vi "stage_xy_gui.vi"(10 "enable":refnum<vi>, 11 "conn_xyz_in":T2) -> (0 "position_y":dbl format="%#.3f", 1 "position_x":dbl format="%#.3f", 3 "conn_xyz_out":T1)   [LabVIEW 2014]
uses:
  D:/felipe/Microscope/Software/Tools/Stage_xyz/Dll/Newport.CONEXCC.CommandInterface.dll
  Tools/Stage_xyz/Dll/Newport.CONEXCC.CommandInterface.dll
  <vilib>/Utility/miscctls.llb/LVPointDoubleTypeDef.ctl
  GLOBAL_VAR.vi
panel:
  in  "Tab Control":enum32{"Position", "Status"}(tab)
  in  "y_val":dbl caption="Y:" min=0.0 max=11.0 format="%.3g"
  in  "x_val":dbl caption="X:" min=0.0 max=11.0 format="%.3g"
  out "xy_position":cluster{"X":dbl, "Y":dbl}[](graph)
  in  "stop_move":bool
  out "current_speed_y":dbl=0.4 caption="Y:" min=0.0 max=25.0 format="%#.3f"
  out "state_y":u32 caption="Y:"
  out "state_x":u32 caption="X:"
  out "current_speed_x":dbl=0.4 caption="X:" min=0.0 max=25.0 format="%#.3f"
  # "State :"
  # "Position :"
  # "Speed :"
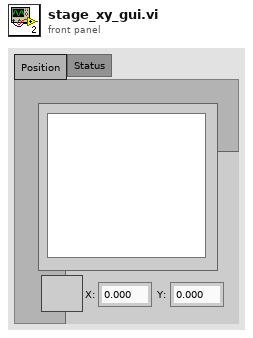
[diagram p1: front panel]
types:
  T1 = cluster{"conn_x_out":refnum<k24>, "conn_y_out":refnum<k24>, "conn_z_out":refnum<k24>}
  T2 = cluster{"conn_x_in":refnum<k24>, "conn_y_in":refnum<k24>, "conn_z_in":refnum<k24>}
  T3 = typedef "LVPointDoubleTypeDef.ctl" = cluster{"X":dbl, "Y":dbl}
  T4 = enum16{"Standby", "Goto", "Stop", "Status", "Goto_z"}
  T5 = cluster{"controllerState":u32, "controllerState":u32, "controllerState":u32}
  T6 = cluster{"Velocity":dbl, "Velocity":dbl, "Velocity":dbl}
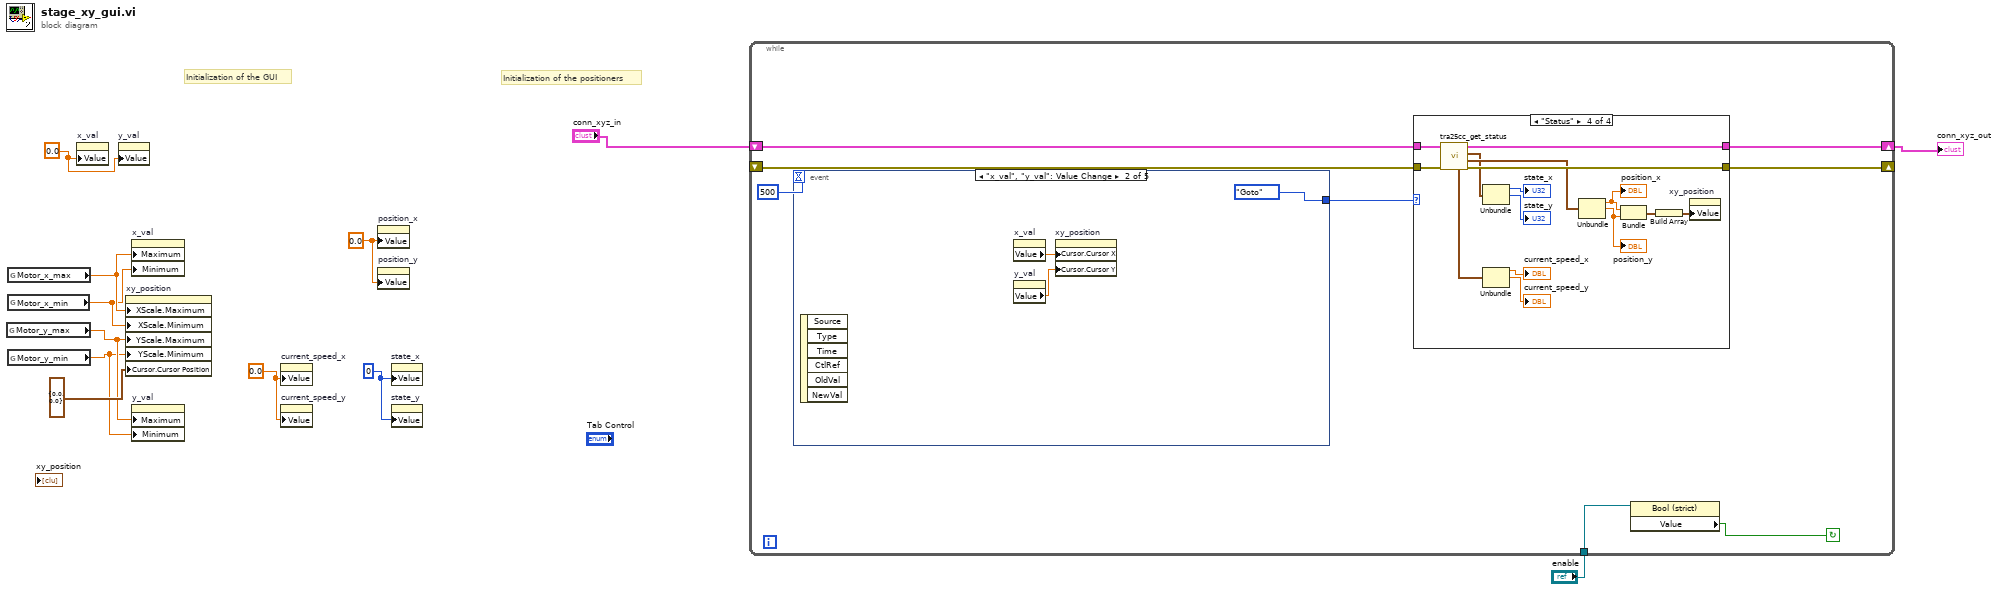
[diagram p0: block diagram]
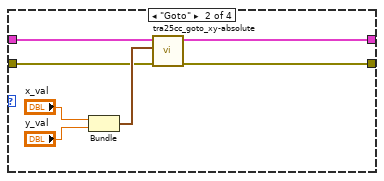
[diagram p3: hidden frame]
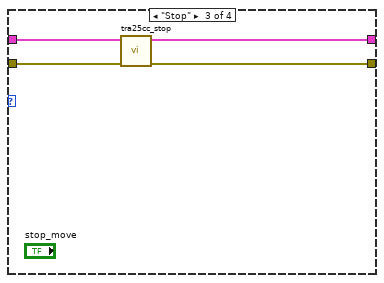
[diagram p4: hidden frame]
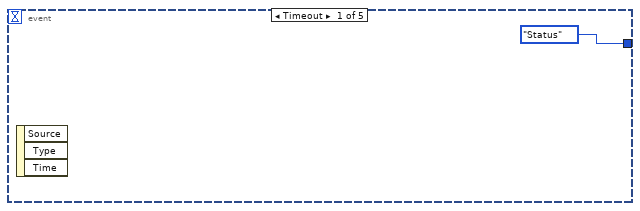
[diagram p5: hidden frame]
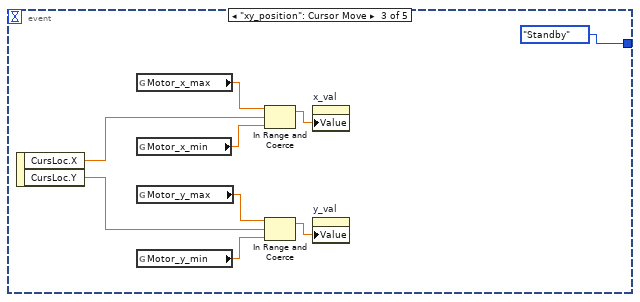
[diagram p6: hidden frame]
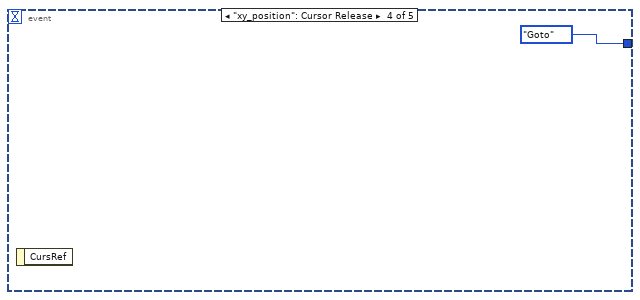
[diagram p7: hidden frame]
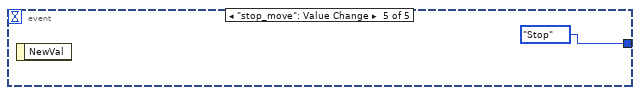
[diagram p8: hidden frame]
diagram:
  w8 = 0.0 ("position_x")
  w9 = u32 0 ("state_x")
  w10 = 0.0 ("current_speed_x")
  w12 = 0.0 ("x_val")
  # "Initialization of the positioners"
  # "Initialization of the GUI"
  n1 = global read "GLOBAL_VAR.vi" "Motor_y_max"() -> (w5:dbl)
  n2 = global read "GLOBAL_VAR.vi" "Motor_x_max"() -> (w7:dbl)
  n3 = global read "GLOBAL_VAR.vi" "Motor_x_min"() -> (w6:dbl)
  n4 = global read "GLOBAL_VAR.vi" "Motor_y_min"() -> (w4:dbl)
  n5 = property on="x_val" class="DigNum (strict)"("Value"=w12) -> ()  [unwired: 2 in, 2 out]
  n6 = property on="y_val" class="DigNum (strict)"("Value"=w12) -> ()  [unwired: 2 in, 2 out]
  n7 = property on="xy_position" class="XYGraph (strict)"("XScale.Maximum"=w7, "XScale.Minimum"=w6, "YScale.Maximum"=w5, "YScale.Minimum"=w4, "Cursor.Cursor Position"=T3 {"X"=0.0, "Y"=0.0}) -> ()  [unwired: 2 in, 2 out]
  n8 = property on="x_val" class="DigNum (strict)"("Maximum"=w7, "Minimum"=w6) -> ()  [unwired: 2 in, 2 out]
  n9 = property on="y_val" class="DigNum (strict)"("Maximum"=w5, "Minimum"=w4) -> ()  [unwired: 2 in, 2 out]
  n10 = property on="current_speed_x" class="DigNum (strict)"("Value"=w10) -> ()  [unwired: 2 in, 2 out]
  n11 = property on="current_speed_y" class="DigNum (strict)"("Value"=w10) -> ()  [unwired: 2 in, 2 out]
  n12 = property on="position_x" class="DigNum (strict)"("Value"=w8) -> ()  [unwired: 2 in, 2 out]
  n13 = property on="position_y" class="DigNum (strict)"("Value"=w8) -> ()  [unwired: 2 in, 2 out]
  n14 = property on="state_x" class="DigNum (strict)"("Value"=w9) -> ()  [unwired: 2 in, 2 out]
  n15 = property on="state_y" class="DigNum (strict)"("Value"=w9) -> ()  [unwired: 2 in, 2 out]
  n16 = while {
    shift-right: [w17] -> w2
    shift-left: "conn_xyz_in" -> [w18]
    shift-right: [w16] -> _
    shift-left: _ -> [w19]
    tunnel: "enable" -> [w13]
    stop <- w14 continue-if-true
    n17 = event shown="[1] \"x_val\", \"y_val\": Value Change" {
      selector: _ -> [_ _ _ _ _]
      dyn-events: _ -> [_ _ _ _ _]
      timeout: 500 -> [_ _ _ _ _]
      tunnel: [T4."Status" T4."Goto" T4."Standby" T4."Goto" T4."Stop"] -> w20
      event Timeout {
        n18 = event-data() -> ()  [unwired: 1 in, 3 out]
      }
      event "x_val", "y_val": Value Change {
        n19 = event-data() -> ()  [unwired: 1 in, 6 out]
        n20 = property on="x_val" class="DigNum (strict)"() -> ("Value"=w52:dbl)  [unwired: 2 in, 2 out]
        n21 = property on="y_val" class="DigNum (strict)"() -> ("Value"=w51:dbl)  [unwired: 2 in, 2 out]
        n22 = property on="xy_position" class="XYGraph (strict)"("Cursor.Cursor X"=w52, "Cursor.Cursor Y"=w51) -> ()  [unwired: 2 in, 2 out]
      }
      event "xy_position": Cursor Move {
        n23 = event-data() -> ("CursLoc.X"=w59:dbl, "CursLoc.Y"=w58:dbl)  [unwired: 1 in]
        n24 = global read "GLOBAL_VAR.vi" "Motor_x_max"() -> (w56:dbl)
        n25 = global read "GLOBAL_VAR.vi" "Motor_x_min"() -> (w55:dbl)
        n26 = global read "GLOBAL_VAR.vi" "Motor_y_max"() -> (w54:dbl)
        n27 = global read "GLOBAL_VAR.vi" "Motor_y_min"() -> (w53:dbl)
        n28 = In Range and Coerce(upper limit=w56, x=w59, lower limit=w55) -> (coerced(x)=w61:dbl)  [unwired: 1 out]
        n29 = In Range and Coerce(upper limit=w54, x=w58, lower limit=w53) -> (coerced(x)=w60:dbl)  [unwired: 1 out]
        n30 = property on="x_val" class="DigNum (strict)"("Value"=w61) -> ()  [unwired: 2 in, 2 out]
        n31 = property on="y_val" class="DigNum (strict)"("Value"=w60) -> ()  [unwired: 2 in, 2 out]
      }
      event "xy_position": Cursor Release {
        n32 = event-data() -> ()  [unwired: 1 in, 1 out]
      }
      event "stop_move": Value Change {
        n33 = event-data() -> ()  [unwired: 1 in, 1 out]
      }
    }
    n34 = case shown="\"Status\"" w20 {
      tunnel: [w22 w26 w32 w46] -> w17
      tunnel: [w21 w23 w30 w45] -> w16
      tunnel: w18 -> [w22 w27 w33 w48]
      tunnel: w19 -> [w21 w24 w31 w47]
      frame "Standby", Default {
      }
      frame "Goto" {
        n35 = Bundle("x_val"="x_val", "y_val"="y_val") -> (w25:cluster{"x_val":dbl, "y_val":dbl})  [unwired: 1 in]
        n36 = call "tra25cc_goto_xy-absolute.vi"("error in (no error)"=w24, "xy_val_mm"=w25, "conn_xyz_in"=w27) -> ("error out"=w23:errorcluster, "conn_xyz_out"=w26:T1)  [unwired: 7 in]
      }
      frame "Stop" {
        n37 = call "tra25cc_stop.vi"("error in (no error)"=w31, "conn_xyz_in"=w33) -> ("error out"=w30:errorcluster, "conn_xyz_out"=w32:T1)  [unwired: 8 in]
      }
      frame "Status" {
        n38 = call "tra25cc_get_status.vi"("error in (no error)"=w47, "conn_xyz_in"=w48) -> ("error out"=w45:errorcluster, "position_xyz"=w43:cluster{"pos_x":dbl, "pos_y":dbl, "pos_z":dbl}, "state_xyz"=w38:T5, "conn_xyz_out"=w46:T1, "current_speed_xyz"=w44:T6)  [unwired: 5 in]
        n39 = Unbundle(w38) -> ("controllerState"=→"state_x":u32, "controllerState"=→"state_y":u32)  [unwired: 1 out]
        n40 = Unbundle(w44) -> ("Velocity"=→"current_speed_x":dbl, "Velocity"=→"current_speed_y":dbl)  [unwired: 1 out]
        n41 = Unbundle(w43) -> ("pos_x"=w41:dbl, "pos_y"=w40:dbl)  [unwired: 1 out]
        "position_x" <- w41
        "position_y" <- w40
        n42 = Bundle("pos_x"=w41, "pos_y"=w40) -> (w42:cluster{"pos_x":dbl, "pos_y":dbl})  [unwired: 1 in]
        n43 = Build Array(w42) -> (w39:cluster{"pos_x":dbl, "pos_y":dbl}[])
        n44 = property on="xy_position" class="XYGraph (strict)"("Value"=w39) -> ()  [unwired: 2 in, 2 out]
      }
    }
    n45 = property class="Bool (strict)"(reference=w13) -> ("Value"=w14:bool)  [unwired: 1 in, 2 out]
  }
  "conn_xyz_out" <- w2
